vi "Hardware Aquisition.vi"(8 "error in (no error)":errorcluster, 10 "Hardware Paramentes In":T2 {"Units" items=["us", "ms"]; "Gain1 (dB)" min=-5 max=45 step=1; "Power Level" max=1023 step=1; "Phase" max=270 step=90; "Frequency" min=1.0 format="%^#_6e"; "CuttOff Freq2[MHz]" min=1 max=30 step=1; "CuttOff Freq1[MHz]" min=1 max=30 step=1; "Gain2 (dB)" min=-5 max=45 step=1; "Time Between Points" min=0.0 step=1.0; "Number Samples" step=1}, 11 "class objects in":T1) -> (0 "error out":errorcluster, 3 "class objects out":T1)   [LabVIEW 2011]
uses:
  Controls/Hardware Control.ctl
  Controls/Class Objects.ctl
  Modules/File/Configuration/Configuration.lvclass
  Modules/Hardware/Power Supply/Power Supply.lvclass
  Modules/Hardware/NMR/NMR.lvclass
  Modules/File/TDMS/TDMS.lvclass
  Controls/User Interface Action.ctl
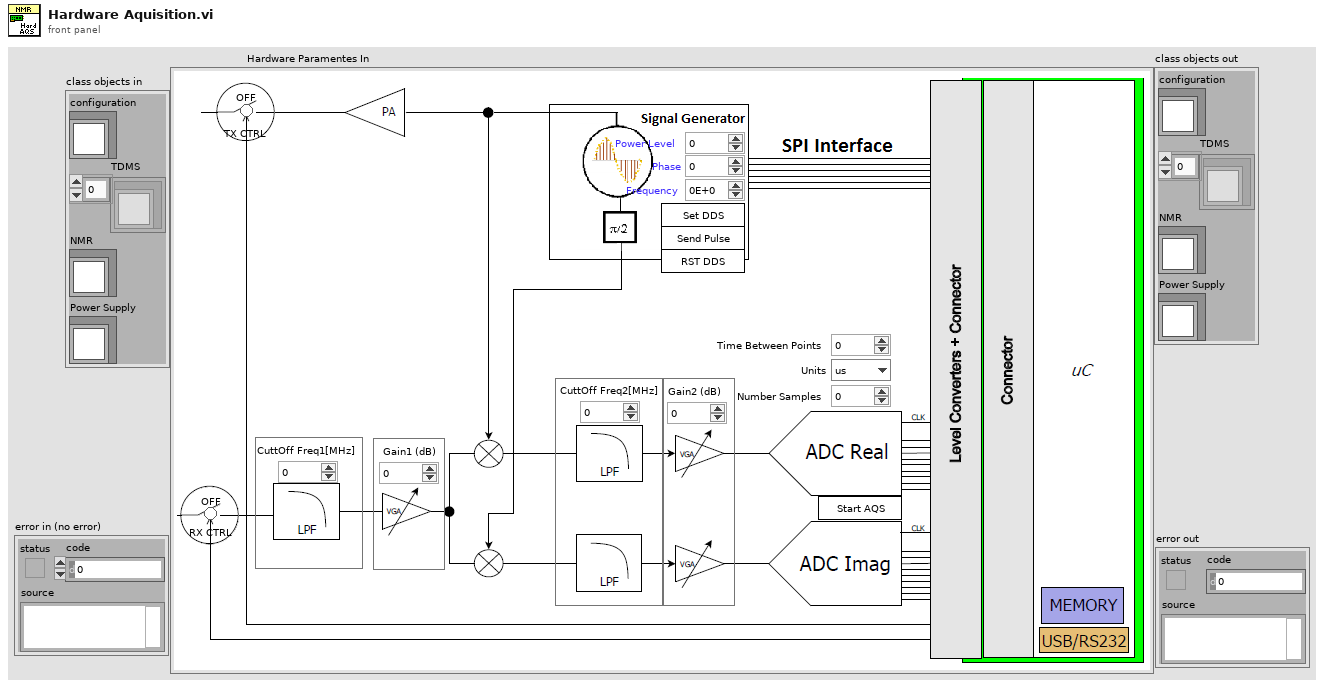
[diagram p1: front panel]
types:
  T1 = typedef "Class Objects.ctl" = cluster{"configuration":refnum<class "Configuration.lvclass">, "TDMS":refnum<class "TDMS.lvclass">[], "Power Supply":refnum<class "Power Supply.lvclass">, "NMR":refnum<class "NMR.lvclass">}
  T2 = typedef "Hardware Control.ctl" = cluster{"Number Samples":u16, "Time Between Points":dbl, "Gain2 (dB)":i8, "CuttOff Freq1[MHz]":u8, "CuttOff Freq2[MHz]":u8, "Frequency":dbl, "Phase":u16, "Power Level":u16, "Send Pulse":bool, "Reset DDS":bool, "TX CTRL":bool, "RX CTRL":bool, "Gain1 (dB)":i8, "Set DDS":bool, "Start AQS":bool, "Units":u8}
  T3 = typedef "User Interface Action.ctl" = enum16{"Initialize", "Update Real Channel", "Update Imag Channel", "Update Re/Im channel @ Hardware Ctrl", "Pulse Sequence", "Visibility Front Panel Controls", "Report Custom Errors", "Set Pulse Sequence Type", "Update Pulse Timings", "Update Transfer Time", "Update Status Bar", "Set Sequence Progress", "Set 90 Degree Pulse Sequence Params", "Set CMPG Pulse Sequence Parms", "Set T1 Pulse Sequence Params", "Stop"}
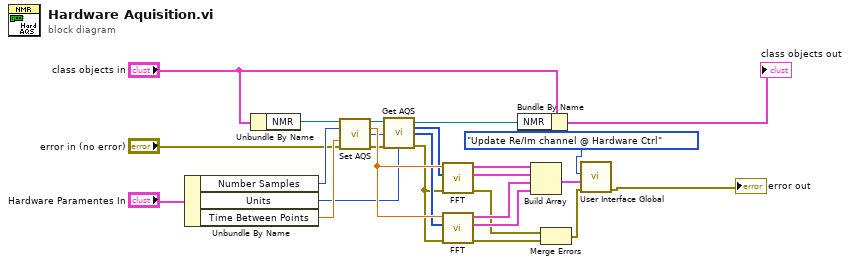
[diagram p0: block diagram]
diagram:
  n1 = Unbundle By Name("Hardware Paramentes In") -> ("Number Samples"=w6:u16, "Units"=w7:u8, "Time Between Points"=w16:dbl)
  n2 = Unbundle By Name("class objects in") -> ("NMR"=w1:refnum<class "NMR.lvclass">)
  n3 = call-dynamic "Set AQS.vi"("NMR in"=w1, "Number Samples"=w6, "Units"=w7, "Time Between Points"=w16, "error in (no error)"="error in (no error)") -> ("NMR out"=w8:refnum<class "NMR.lvclass">, "Real Time"=w17:ext, "error out"=w9:errorcluster)  [unwired: 7 in, 1 out]
  n4 = call-dynamic "Get AQS.vi"("NMR in"=w8, "error in (no error)"=w9) -> ("NMR out"=w10:refnum<class "NMR.lvclass">, "Real Data"=w11:i32[], "Imag Data"=w13:i32[], "error out"=w12:errorcluster)  [unwired: 10 in]
  n5 = call "FFT.vi"("error in (no error)"=w12, "Input Array"=w11, "Delay Sample"=w17) -> ("error out"=w14:errorcluster, "Time Graph"=w18:cluster{"magnitude":dbl[], dbl[]}, "FFT Graph"=w24:cluster{"magnitude":dbl[], dbl[]})  [unwired: 6 in]
  n6 = call "FFT.vi"("error in (no error)"=w12, "Input Array"=w13, "Delay Sample"=w17) -> ("error out"=w15:errorcluster, "Time Graph"=w25:cluster{"magnitude":dbl[], dbl[]}, "FFT Graph"=w19:cluster{"magnitude":dbl[], dbl[]})  [unwired: 6 in]
  n7 = Bundle By Name(cluster="class objects in", "NMR"=w10) -> (→"class objects out":T1)
  n8 = Build Array(w24, w18, w19, w25) -> (w21:cluster{"magnitude":dbl[], dbl[]}[])
  n9 = Merge Errors(w14, w15) -> (w22:errorcluster)
  n10 = call "User Interface Global.vi"("error in"=w22, "data1"=w21, "action"=User_Interface_Action."Update Re/Im channel @ Hardware Ctrl") -> ("error out"=→"error out":errorcluster)  [unwired: 8 in]
